vi "get apdm file version.vi"(10 "version":u32(ring) items=["APDM_FILE_VERSION_UNKNOWN", "APDM_FILE_VERSION_0000", "APDM_FILE_VERSION_0001", "APDM_FILE_VERSION_0002", "APDM_FILE_VERSION_0003", "APDM_FILE_VERSION_0004", "APDM_FILE_VERSION_0005", "APDM_FILE_VERSION_0006", "APDM_FILE_VERSION_0007", "APDM_FILE_VERSION_2001"], 11 "filepath":string) -> (2 "version out":u32(ring) items=["APDM_FILE_VERSION_UNKNOWN", "APDM_FILE_VERSION_0000", "APDM_FILE_VERSION_0001", "APDM_FILE_VERSION_0002", "APDM_FILE_VERSION_0003", "APDM_FILE_VERSION_0004", "APDM_FILE_VERSION_0005", "APDM_FILE_VERSION_0006", "APDM_FILE_VERSION_0007", "APDM_FILE_VERSION_2001"], 3 "function return":i32)   [LabVIEW 2019, in "apdm.lvlib"]
doc: "APDM_EXPORT int apdm_get_apdm_file_version(const char * filepath, apdm_file_version_t *version);"
uses:
  apdm.lvlib
  Lee Lab/CP FES Walking 2018/Code/Working/LabVIEW/apdm.dll
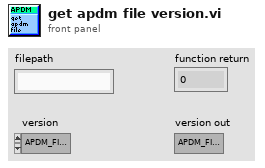
[diagram p1: front panel]
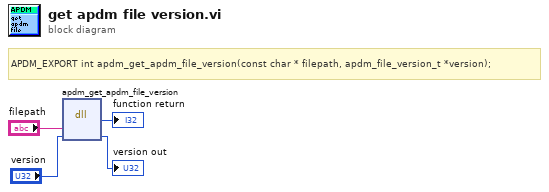
[diagram p0: block diagram]
diagram:
  # "APDM_EXPORT int apdm_get_apdm_file_version(const char * filepath, apdm_file_version_t *version);"
  n1 = dll-call lib="C:/Users/jfalesi/Dropbox/Lee Lab/CP FES Walking 2018/Code/Working/LabVIEW/apdm.*" fn="apdm_get_apdm_file_version"("filepath"="filepath", "version"="version") -> (→"function return":i32, "version"=→"version out":u32)  [unwired: 4 in, 2 out]
